vi "cleanup.vi"(2 "error in":errorcluster, 3 "Configuration":T1) -> (0 "error out":errorcluster)   [LabVIEW 2012]
uses:
  configuration.ctl
  asap_calibration.ctl
  <vilib>/Analysis/Matrix/Datatypes/RealMatrix.ctl
  <vilib>/DAQmx/write.llb/DAQmx Write (Digital 1D Bool 1Chan 1Samp).vi
  <vilib>/DAQmx/miscellaneous.llb/DAQmx Fill In Error Info.vi
  <vilib>/Analysis/Matrix/NI_Matrix.lvlib
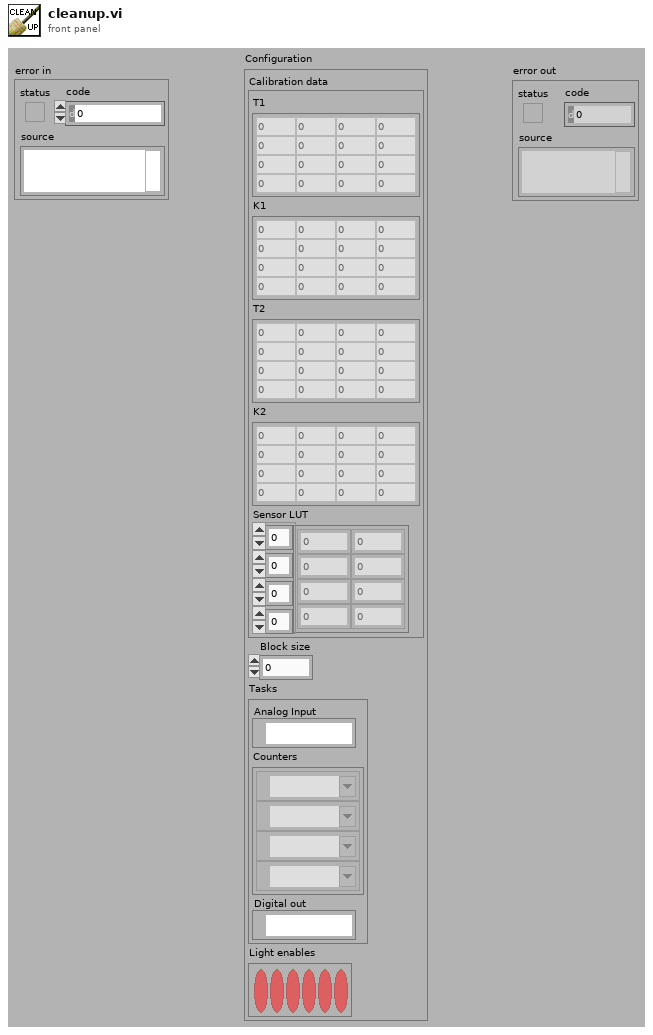
[diagram p1: front panel]
types:
  T1 = typedef "configuration.ctl" = cluster{"Calibration data":T2, "Block size":i32, "Tasks":cluster{"Analog Input":refnum<k21>, "Counters":refnum<k21>[], "Digital out":refnum<k21>}, "Light enables":bool[]}
  T2 = typedef "asap_calibration.ctl" = cluster{"T1":T3, "K1":T3, "T2":T3, "K2":T3, "Sensor LUT":sgl[][][][]}
  T3 = typedef "NI_Matrix.lvlib/RealMatrix.ctl" = dbl[][]
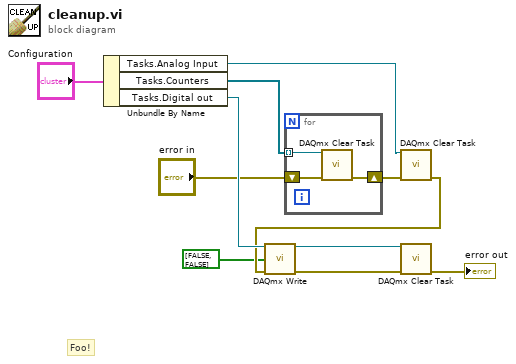
[diagram p0: block diagram]
diagram:
  # "Foo!"
  n1 = Unbundle By Name("Configuration") -> ("Tasks.Analog Input"=w9:refnum<k21>, "Tasks.Counters"=w1:refnum<k21>[], "Tasks.Digital out"=w8:refnum<k21>)
  n2 = for {
    shift-right: [w14] -> w11
    shift-left: "error in" -> [w13]
    tunnel: w1 -> [w12] mode=indexing
    n3 = call <vilib>:"DAQmx Clear Task.vi"("task in"=w12, "error in"=w13) -> ("error out"=w14:errorcluster)  [unwired: 13 out]
  }
  n4 = call <vilib>:"DAQmx Clear Task.vi"("task in"=w9, "error in"=w11) -> ("error out"=w7:errorcluster)  [unwired: 13 out]
  n5 = call-poly <vilib>:"DAQmx Write.vi"("task/channels in"=w8, "data"=bool[] [FALSE, FALSE], "error in"=w7) -> ("task out"=w4:refnum<k21>, "error out"=w3:errorcluster)  [unwired: 1 in, 10 out]
  n6 = call <vilib>:"DAQmx Clear Task.vi"("task in"=w4, "error in"=w3) -> ("error out"=→"error out":errorcluster)  [unwired: 13 out]
